vi "test.vi"() -> ()   [LabVIEW 2020]
uses:
  zlgcan.lvlib
panel:
  out "before substring":string
  out "offset past match":i32
  out "startcan_success? 2":bool
  out "CAN DATA":string
  out "error out 2":errorcluster
  out "status":bool
  out "error out":errorcluster caption="错误输出"
  out "startcan_success?":bool
  in  "can_index":u32
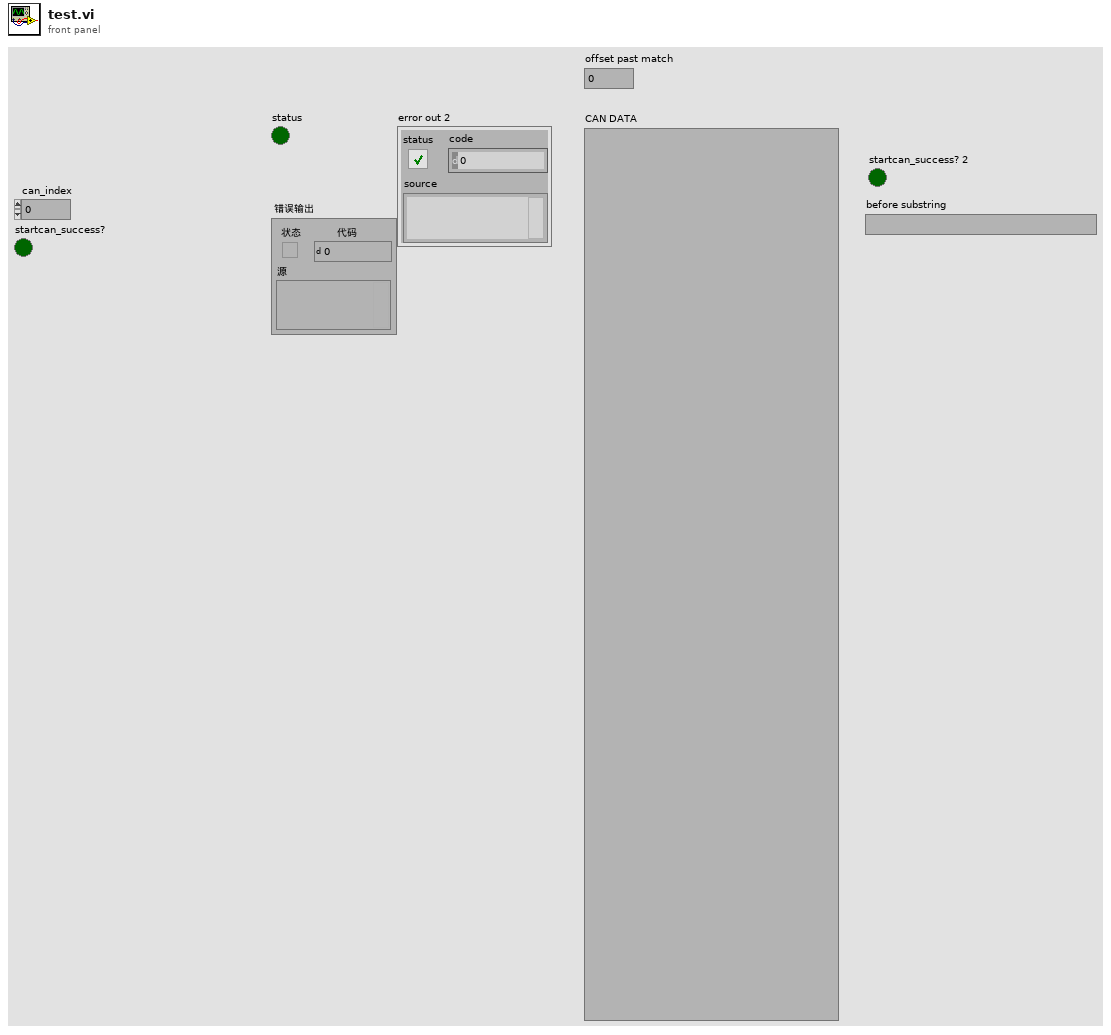
[diagram p1: front panel]
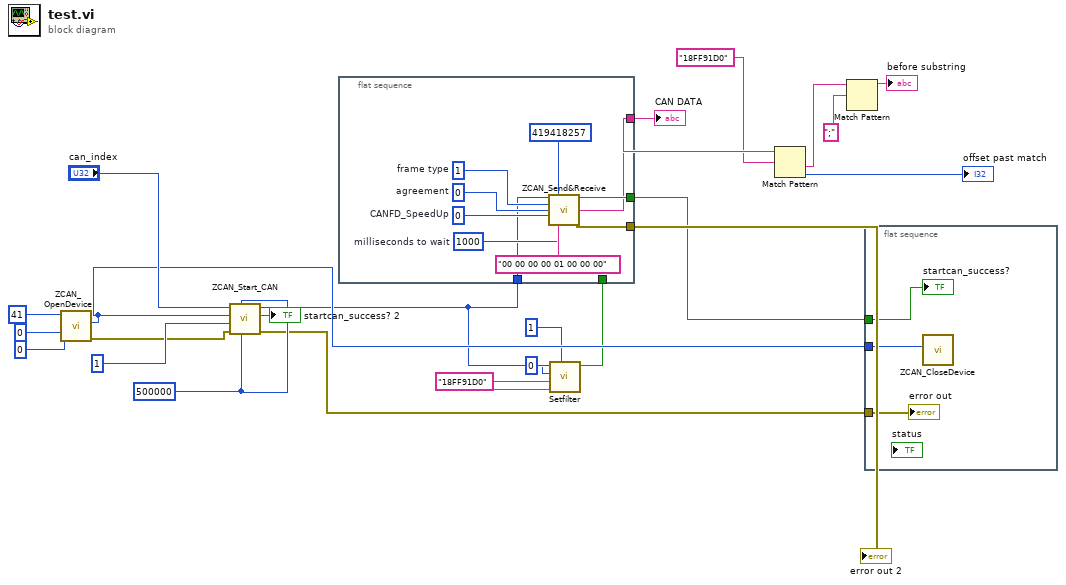
[diagram p0: block diagram]
diagram:
  w2 = "18FF91D0" ("filter_end")
  w21 = u32 500000 ("abitbaud")
  n1 = call "ZCAN_OpenDevice.vi"("reserved"=u32 0, "device_index"=u32 0, "device_type"=u32 41) -> ("error out"=w16:errorcluster, "DEVICE_HANDLE"=w15:u32)  [unwired: 7 in]
  n2 = call "ZCAN_Start_CAN.vi"("abitbaud"=w21, "dbitbaud"=w21, "error in (no error)"=w16, "ResistanceEnable"=u32 1, "device_hande"=w15, "can_index"="can_index") -> ("error out"=w20:errorcluster, "startcan_success?"=→"startcan_success? 2":bool, "can_index_handle(out)"=w4:u32)  [unwired: 3 in]
  n3 = flat-sequence {
    tunnel: [w29] -> w14
    tunnel: [w28] -> w13
    tunnel: [w25] -> w11
    tunnel: w4 -> [w24]
    tunnel: w1 -> [_]
    frame #0 {
      w26 = u32 0  # CANFD_SpeedUp
      w30 = u32 1000  # milliseconds to wait
      w27 = u32 0  # agreement
      w32 = u32 1  # frame type
      n4 = call "ZCAN_Send&Receive.vi"("can_index_handle"=w24, "ID"=u32 419418257, "frame type"=w32, "agreement"=w27, "CANFD_SpeedUp"=w26, "Data"="00 00 00 00 01 00 00 00", "milliseconds to wait"=w30) -> ("status"=w28:bool, "error out"=w29:errorcluster, "CAN DATA"=w25:string)  [unwired: 5 in, 1 out]
    }
  }
  n5 = call "Setfilter.vi"("filter_mode"=u32 1, "filter_start"=w2, "filter_end"=w2, "can_index"=u32 0, "device_handle"=w4) -> ("SetfilterResult"=w1:bool)  [unwired: 5 in]
  n6 = Match Pattern(string=w11, regular expression="18FF91D0") -> (after substring=w7:string, offset past match=→"offset past match":i32)  [unwired: 1 in, 2 out]
  n7 = Match Pattern(string=w7, regular expression=";" ("string")) -> (before substring=→"before substring":string)  [unwired: 1 in, 3 out]
  n8 = flat-sequence {
    tunnel: w13 -> [w36]
    tunnel: w20 -> [w35]
    tunnel: w15 -> [w34]
    frame #0 {
      n9 = call "ZCAN_CloseDevice.vi"("device_handle"=w34) -> ()  [unwired: 9 in, 2 out]
      "startcan_success?" <- w36
      "error out" <- w35
    }
  }
  "error out 2" <- w14
  "CAN DATA" <- w11
